vi "Handle Last Ack Core.vi"(4 "error in (no error)":errorcluster, 6 "Last Ack":refnum<class "Last Ack.lvclass">, 7 "Server in":refnum<class "Server.lvclass">) -> (0 "error out":errorcluster, 3 "Server out":refnum<class "Server.lvclass">)   [LabVIEW 2014, in "Server.lvlib" / "Server.lvclass"]
doc: "(<B>Filename</B>: Actor Framework.lvlib:Actor.lvclass:Handle Last Ack Core.vi)\n\nDefines how the caller actor responds to the Last Ack message from a nested actor. The Last Ack message is the final message a nested actor sends to its caller before it shuts down. The message contains information about the final state of the nested actor.\n\nBy default, this method does nothing except return any error the nested actor sent. A descendant class may override this method to define behavior."
uses:
  Server.lvclass
  <vilib>/ActorFramework/LastAck/Last Ack.lvclass
  Chat Window Model/Chat Window Model Messages/Update Online List Msg/Update Online List Msg.lvclass
  Chat Window Model/Chat Window Model Messages/Update Status Log Msg/Update Status Log Msg.lvclass
  Server Messages/Enable Controls Msg/Enable Controls Msg.lvclass
  <vilib>/ActorFramework/Actor/Actor.lvclass
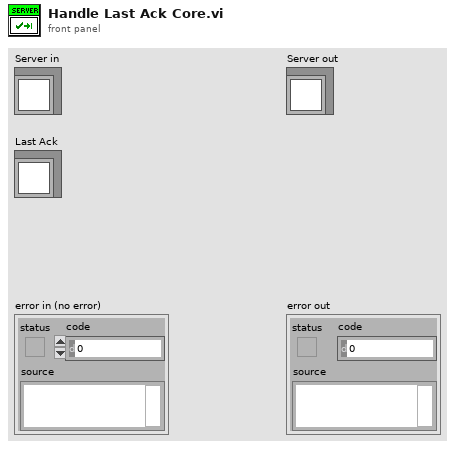
[diagram p1: front panel]
types:
  T1 = enum8{"Enabled", "Disabled", "Disabled and Grayed Out"}
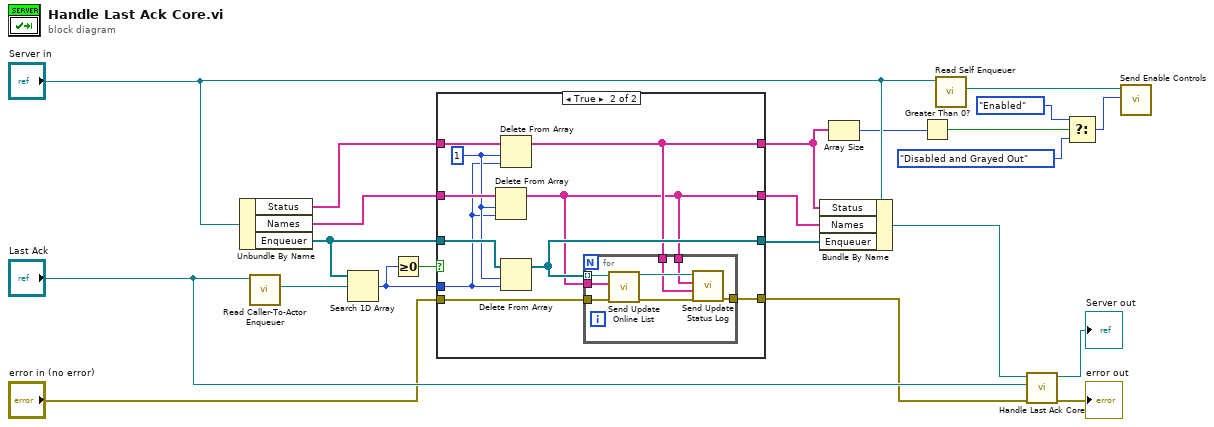
[diagram p0: block diagram]
diagram:
  n1 = Unbundle By Name("Server in") -> ("Status"=w11:string[], "Names"=w13:string[], "Enqueuer"=w18:refnum<class "Message Enqueuer.lvclass">[])
  n2 = call <vilib>:"Read Caller-To-Actor Enqueuer.vi"("Last Ack"="Last Ack") -> ("Caller-to-Actor Enqueuer"=w19:refnum<class "Message Enqueuer.lvclass">)  [unwired: 10 in]
  n3 = Search 1D Array(1D array=w18, element=w19) -> (index of element=w17:i32)  [unwired: 1 in]
  n4 = Greater Or Equal To 0?(x=w17) -> (x >= 0?=w16:bool)
  n5 = case shown="True" w16 {
    tunnel: w18 -> [w26 w36]
    tunnel: w17 -> [_ w31]
    tunnel: [w26 w34] -> w14
    tunnel: w13 -> [w25 w35]
    tunnel: [w25 w29] -> w12
    tunnel: w11 -> [w24 w33]
    tunnel: [w24 w30] -> w6
    tunnel: "error in (no error)" -> [w23 w28]
    tunnel: [w23 w27] -> w9
    frame False {
    }
    frame True {
      w32 = 1 ("length")
      n6 = Delete From Array(array=w35, length=w32, index=w31) -> (array with subset deleted=w29:string[])  [unwired: 1 out]
      n7 = Delete From Array "Delete From Array"(array=w33, length=w32, index=w31) -> (array with subset deleted=w30:string[])  [unwired: 1 out]
      n8 = Delete From Array(array=w36, length=w32, index=w31) -> (array with subset deleted=w34:refnum<class "Message Enqueuer.lvclass">[])  [unwired: 1 out]
      n9 = for {
        tunnel: w34 -> [w43] mode=indexing
        tunnel: w29 -> [w44]
        tunnel: w30 -> [w40]
        tunnel: w29 -> [w39]
        tunnel: w28 -> [w38]
        tunnel: [w37] -> w27
        n10 = call "Send Update Online List.vi"("error in (no error)"=w38, "Online Users"=w44, "Message Enqueuer"=w43) -> ("error out"=w41:errorcluster, "Message Enqueuer out"=w42:refnum<class "Message Enqueuer.lvclass">)  [unwired: 7 in]
        n11 = call "Send Update Status Log.vi"("error in (no error)"=w41, "Status List"=w40, "Names"=w39, "Message Enqueuer"=w42) -> ("error out"=w37:errorcluster)  [unwired: 6 in, 1 out]
      }
    }
  }
  n12 = Bundle By Name(cluster="Server in", "Status"=w6, "Names"=w12, "Enqueuer"=w14) -> (w15:refnum<class "Server.lvclass">)
  n13 = Array Size(array=w6) -> (size(s)=w5:i32)
  n14 = Greater Than 0?(x=w5) -> (x > 0?=w4:bool)
  n15 = call <vilib>:"Read Self Enqueuer.vi"("Actor"="Server in") -> ("Self Enqueuer"=w7:refnum<class "Message Enqueuer.lvclass">)  [unwired: 10 in]
  n16 = call-parent "Handle Last Ack Core.vi"("error in (no error)"=w9, "Last Ack"="Last Ack", "Actor in"=w15) -> ("error out"=→"error out":errorcluster, "Actor out"=→"Server out":refnum<class "Server.lvclass">)  [unwired: 3 in]
  n17 = Select(t=T1."Enabled" ("Disabled"), s=w4, f=T1."Disabled and Grayed Out" ("Disabled")) -> (s? t:f=w3:T1)
  n18 = call "Send Enable Controls.vi"("Disabled"=w3, "Message Enqueuer"=w7) -> ()  [unwired: 8 in, 2 out]
